vi "Node Config.vi"(8 "error in (no error)":errorcluster, 11 "DemoApp in":refnum<class "DemoApp.lvclass">) -> (0 "error out":errorcluster, 2 "Node Config":refnum<class "Node Config.lvclass">, 3 "DemoApp out":refnum<class "DemoApp.lvclass">)   [LabVIEW 2020, in "VolatusDemo.lvlib" / "DemoApp.lvclass"]
uses:
  DemoApp.lvclass
  lv-vecto/Vecto/Node Config/Node Config.lvclass
  lv-vecto/Vecto/Node Config/Node Info.ctl
  lv-vecto/Vecto/Node Config/Discovery Info.ctl
  lv-vecto/Vecto/Node Config/HTTP Server Info.ctl
  DemoApp.lvclass/DemoApp.ctl
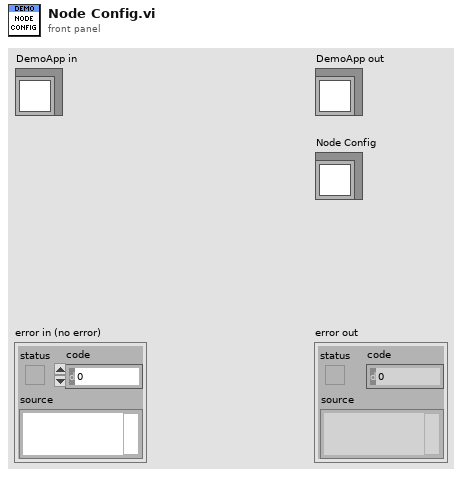
[diagram p1: front panel]
types:
  T1 = typedef "Vecto.lvlib/Node Config.lvclass/HTTP Server Info.ctl" = cluster{"HTTP Port":u16, "Debug":bool}
  T2 = typedef "Vecto.lvlib/Node Config.lvclass/Discovery Info.ctl" = cluster{"Address":string, "Port":u16, "Interval S":dbl, "Bind Address":string}
  T3 = typedef "Vecto.lvlib/Node Config.lvclass/Node Info.ctl" = cluster{"System":string, "Cluster":string, "Name":string, "ID":u32, "Capabilities":string[]}
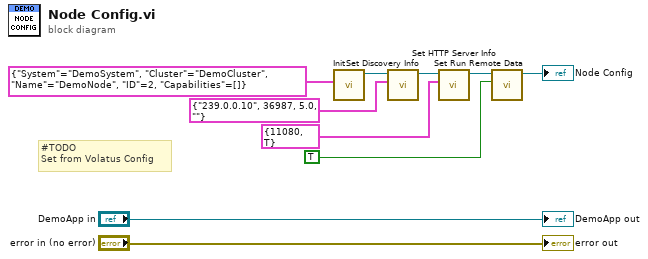
[diagram p0: block diagram]
diagram:
  # "#TODO\nSet from Volatus Config"
  n1 = call "Init.vi"("Node Info"=T3 {"System"="DemoSystem", "Cluster"="DemoCluster", "Name"="DemoNode", "ID"=2, "Capabilities"=[]}) -> ("Node out"=w7:refnum<class "Node Config.lvclass">)  [unwired: 9 in, 1 out]
  n2 = call "Set Discovery Info.vi"("Discovery Info"=T2 {"Address"="239.0.0.10", "Port"=36987, "Interval S"=5.0, "Bind Address"=""}, "Node in"=w7) -> ("Node out"=w5:refnum<class "Node Config.lvclass">)  [unwired: 8 in, 1 out]
  n3 = call "Set HTTP Server Info.vi"("HTTP Server Info"=T1 {"HTTP Port"=11080, "Debug"=TRUE}, "Node Config in"=w5) -> ("Node Config out"=w3:refnum<class "Node Config.lvclass">)  [unwired: 8 in, 1 out]
  n4 = call "Set Run Remote Data.vi"("Run Remote Data"=TRUE, "Node Config in"=w3) -> ("Node Config out"=→"Node Config":refnum<class "Node Config.lvclass">)  [unwired: 8 in, 1 out]
  "error out" <- "error in (no error)"
  "DemoApp out" <- "DemoApp in"
